vi "发送数据记录到文档(子VI).vi"(7 "错误输入":errorcluster, 10 "数组":string[](array[string])) -> (0 "错误输出":errorcluster)   [LabVIEW 2016]
uses:
  <vilib>/Utility/sysdir.llb/System Directory Type.ctl
panel:
  out "路径":path
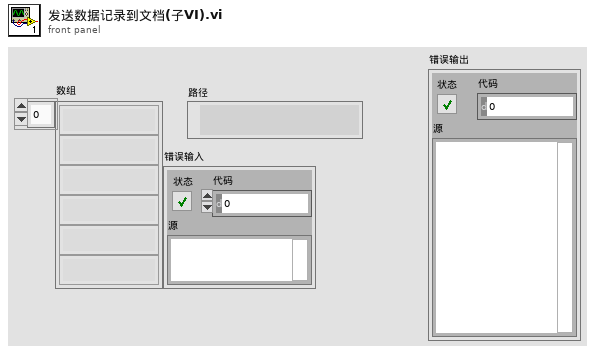
[diagram p1: front panel]
types:
  T1 = typedef "System Directory Type.ctl" = i32
  T2 = enum16{"open", "replace", "create", "open or create", "replace or create", "replace or create with confirmation"}
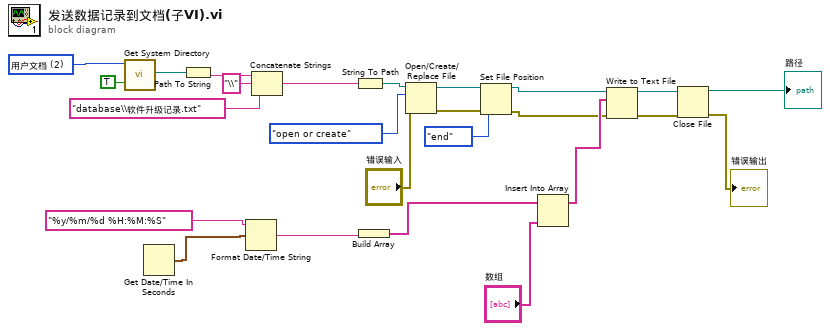
[diagram p0: block diagram]
diagram:
  w16 = T1 2 items=["用户目录"=0, "用户桌面"=1, "用户文档"=2, "用户应用程序数据"=3, "用户设置"=4, "用户临时目录"=5, "公共文档"=6, "公共应用程序数据"=7, "公共设置"=8, "公共缓存"=13, "系统核心库"=9, "系统安装库"=10, "应用程序文件"=11, "启动盘根目录"=12] ("system directory type")
  n1 = call <vilib>:"Get System Directory.vi"("create directory if not found? (F)"=TRUE, "system directory type"=w16) -> ("system directory"=w14:path)  [unwired: 9 in]
  n2 = Get Date/Time In Seconds() -> (seconds since 1Jan1904=w4:timestamp)
  n3 = Path To String(path=w14) -> (string=w13:string)
  n4 = Format Date/Time String(time format string (%c)="%y/%m/%d %H:%M:%S" ("时间格式字符串(%c)"), seconds (now)=w4) -> (date/time string=w1:string)  [unwired: 1 in]
  n5 = Concatenate Strings(w13, "\\" ("字符串"), "database\\软件升级记录.txt" ("字符串")) -> (w10:string)
  n6 = String To Path(string=w10) -> (path=w21:path)
  n7 = Build Array(w1) -> (w2:string[])
  n8 = Open/Create/Replace File(file path (use dialog)=w21, error in="错误输入", operation (0:open)=T2."open or create" ("操作(0:open)")) -> (refnum out=w9:refnum<file>, error out=w8:errorcluster)  [unwired: 3 in, 1 out]
  n9 = Set File Position(refnum=w9, from (0:start)=enum16{"start", "end", "current"}."end" ("自（0:起始）"), error in=w8) -> (refnum out=w7:refnum<file>, error out=w6:errorcluster)  [unwired: 1 in]
  n10 = Insert Into Array(array=w2, new element="数组") -> (w19:string[])  [unwired: 1 in]
  n11 = Write to Text File(file (use dialog)=w7, text=w19, error in=w6) -> (refnum out=w24:refnum<file>, error out=w25:errorcluster)  [unwired: 1 in, 1 out]
  n12 = Close File(refnum=w24, error in=w25) -> (path=→"路径":path, error out=→"错误输出":errorcluster)
